vi "Brownian Motion.vi"(7 "Data":T1) -> (0 "Simulation Objects":refnum<class "SimulationObject.lvclass">[](array[class]), 1 "Cell Size":i16, 2 "Gravity Vector out":refnum<class "Vector2.lvclass">, 3 "Background Color out":u32(colorbox))   [LabVIEW 2022 SP3]
uses:
  Engine/Math/Vector2/Vector2.lvclass
  Engine/Objects/SimulationObject/SimulationObject.lvclass
  Engine/Objects/SimulationObject/SimulationObject.lvclass/SimulationObject.ctl
  Engine/Objects/Components/PhysicsComponent/PhysicsComponent.lvclass/PhysicsComponent.ctl
  Engine/Math/Vector2/Vector2.lvclass/Vector2.ctl
  <vilib>/numeric/Random Number (Range) I64.vi
  Engine/Math/Vector2/Read x.vi
  Engine/Math/Vector2/Read y.vi
  <vilib>/numeric/sub_Random U32.vi
  Engine/Objects/Shapes/CircleShape/CircleShape.lvclass
  D:/Programowanie/Studia/Labview/CollisionSimulator/Project/Engine/Objects/Shapes/Shapeable/Shapeable.lvclass
  Engine/Objects/Components/PhysicsComponent/PhysicsComponent.lvclass
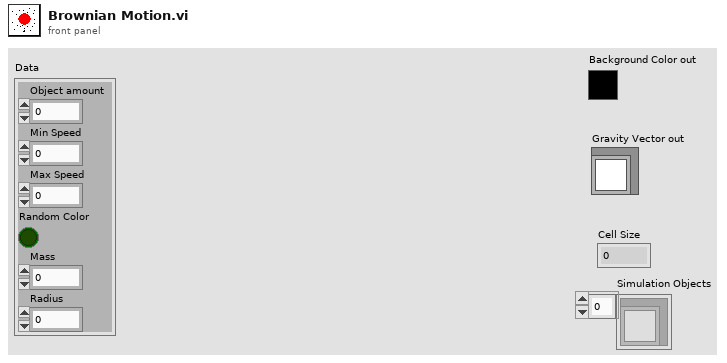
[diagram p1: front panel]
types:
  T1 = cluster{"Object amount":i16, "Min Speed":dbl, "Max Speed":dbl, "Random Color":bool, "Mass":dbl, "Radius":i16}
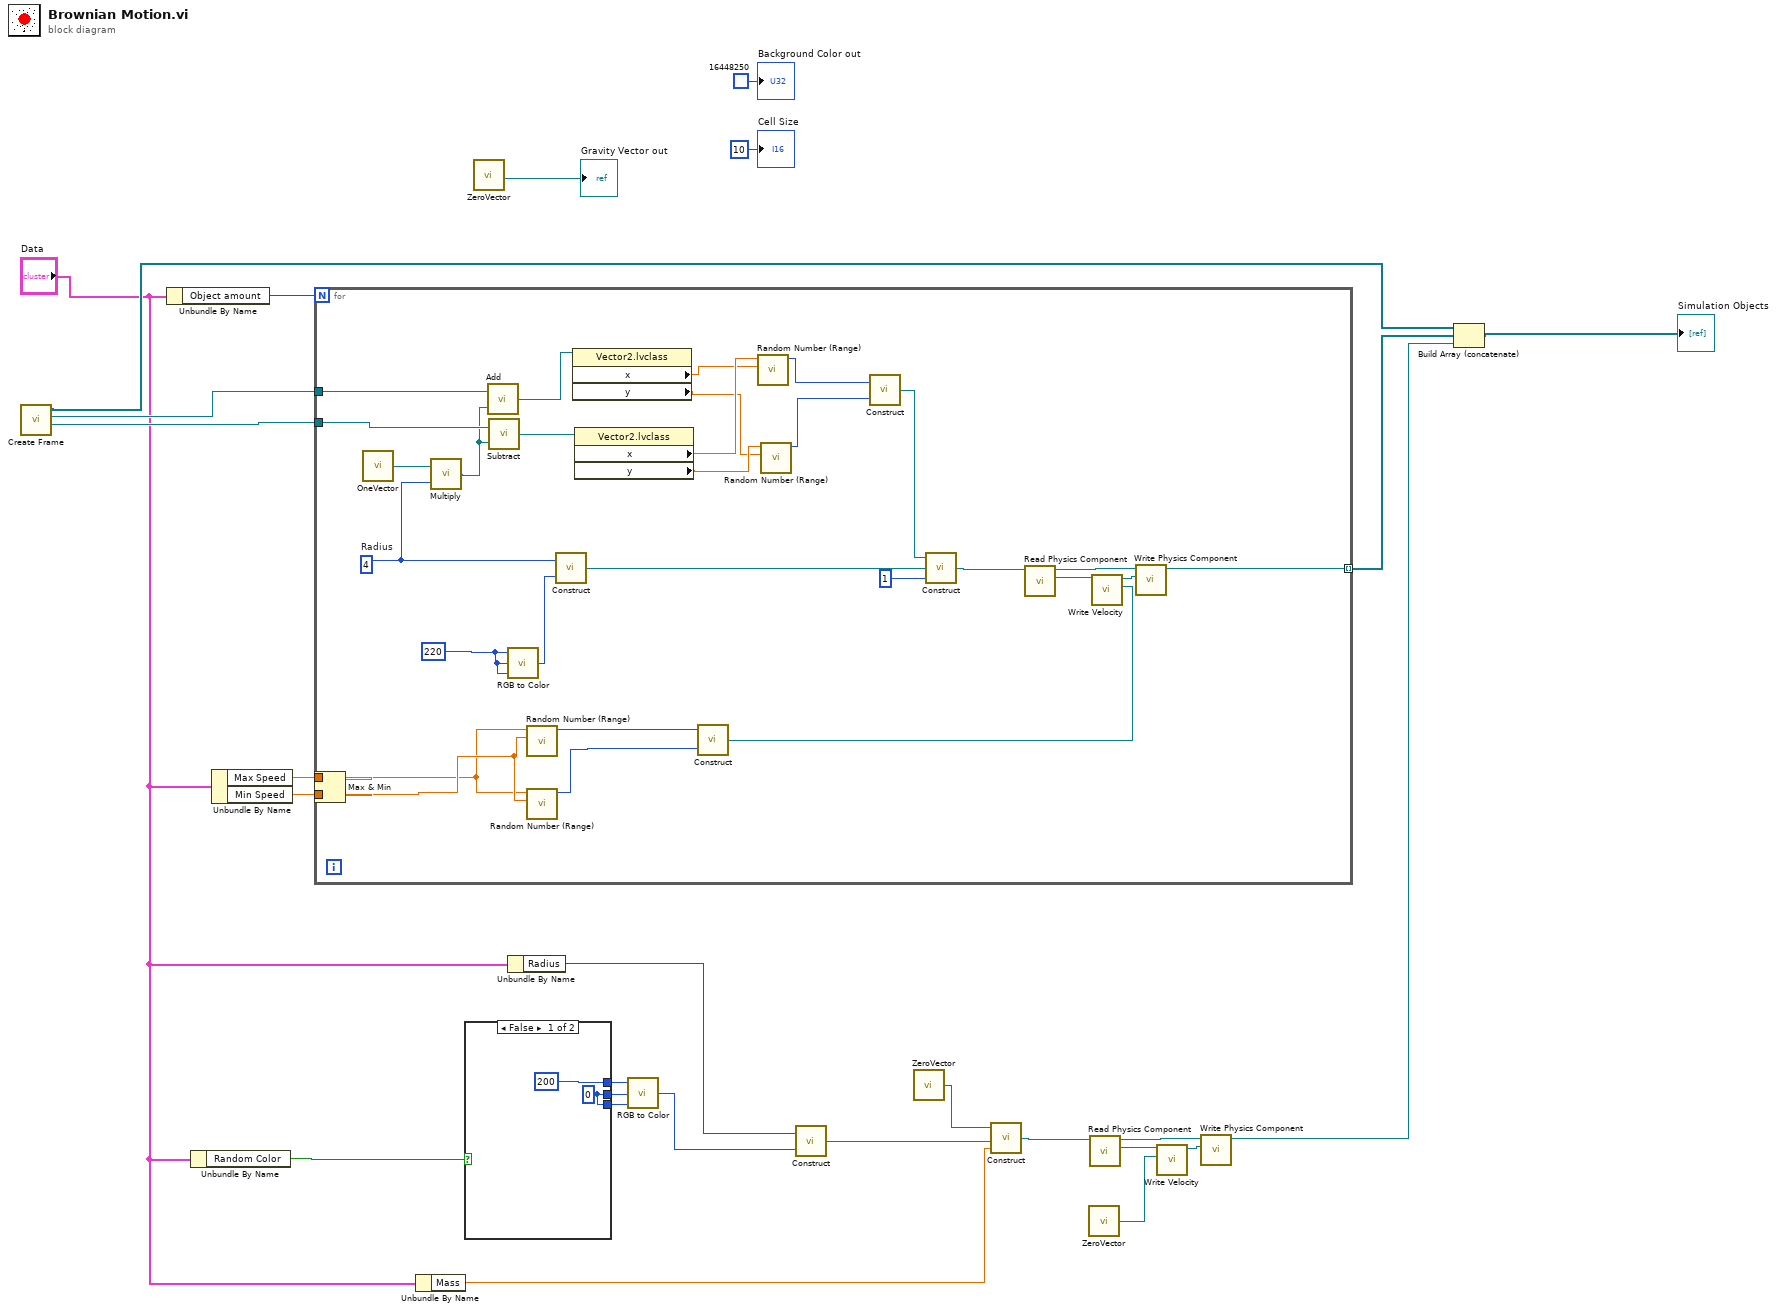
[diagram p0: block diagram]
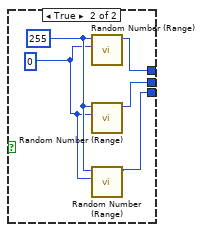
[diagram p2: hidden frame]
diagram:
  n1 = call "Create Frame.vi"() -> ("Max Available Position"=w25:refnum<class "Vector2.lvclass">, "Min Available Position"=w26:refnum<class "Vector2.lvclass">, "Simulation Objects"=w20:refnum<class "SimulationObject.lvclass">[])  [unwired: 4 in, 1 out]
  n2 = Unbundle By Name("Data") -> ("Object amount"=w27:i16)
  n3 = Unbundle By Name("Data") -> ("Random Color"=w13:bool)
  n4 = Unbundle By Name("Data") -> ("Max Speed"=w24:dbl, "Min Speed"=w23:dbl)
  n5 = Max & Min(x=w24, y=w23) -> (max(x,y)=w22:dbl, min(x,y)=w21:dbl)
  n6 = for {
    N: w27 -> [_]
    tunnel: w26 -> [w39]
    tunnel: w25 -> [w49]
    tunnel: w21 -> [w42]
    tunnel: w22 -> [w41]
    tunnel: [w40] -> w19 mode=indexing
    w30 = u8 220 ("R")
    w48 = 4  # Radius
    n7 = call "OneVector.vi"() -> ("One Vector"=w38:refnum<class "Vector2.lvclass">)
    n8 = call "Multiply.vi"("Scalar"=w48, "Vector in"=w38) -> ("Vector out"=w37:refnum<class "Vector2.lvclass">)
    n9 = call "Add.vi"("Vec2 b in"=w37, "Vec2 a in"=w39) -> ("Vec2 out"=w36:refnum<class "Vector2.lvclass">)
    n10 = call "Subtract.vi"("Vec2 b in"=w37, "Vec2 a in"=w49) -> ("Vec2 out"=w35:refnum<class "Vector2.lvclass">)
    n11 = call <vilib>:"RGB to Color.vi"("B"=w30, "G"=w30, "R"=w30) -> ("Color"=w51:u32)
    n12 = call-poly <vilib>:"Random Number (Range).vi"("lower bound (-100)"=w42, "upper bound (100)"=w41) -> ("number"=w44:i64)  [unwired: 9 in]
    n13 = call-poly <vilib>:"Random Number (Range).vi"("lower bound (-100)"=w42, "upper bound (100)"=w41) -> ("number"=w43:i64)  [unwired: 9 in]
    n14 = call "Construct.vi"("Color"=w51, "Radius"=w48) -> ("CircleShape out"=w50:refnum<class "CircleShape.lvclass">)
    n15 = property class="Vector2.lvclass"(reference=w36) -> ("x"=w33:sgl, "y"=w31:sgl)  [unwired: 1 in, 2 out]
    n16 = property class="Vector2.lvclass"(reference=w35) -> ("x"=w34:sgl, "y"=w32:sgl)  [unwired: 1 in, 2 out]
    n17 = call "Construct.vi"("y"=w43, "x"=w44) -> ("Vec2 out"=w52:refnum<class "Vector2.lvclass">)
    n18 = call-poly <vilib>:"Random Number (Range).vi"("lower bound (-100)"=w33, "upper bound (100)"=w34) -> ("number"=w47:i64)  [unwired: 9 in]
    n19 = call-poly <vilib>:"Random Number (Range).vi"("lower bound (-100)"=w31, "upper bound (100)"=w32) -> ("number"=w46:i64)  [unwired: 9 in]
    n20 = call "Construct.vi"("y"=w46, "x"=w47) -> ("Vec2 out"=w57:refnum<class "Vector2.lvclass">)
    n21 = call "Construct.vi"("Mass"=i64 1 ("number"), "Shape in"=w50, "Local Position in"=w57) -> ("Simulation Object out"=w56:refnum<class "SimulationObject.lvclass">)
    n22 = call "Read Physics Component.vi"("SimulationObject in"=w56) -> ("Physics Component out"=w53:refnum<class "PhysicsComponent.lvclass">, "SimulationObject out"=w55:refnum<class "SimulationObject.lvclass">)  [unwired: 8 in, 1 out]
    n23 = call "Write Velocity.vi"("Velocity in"=w52, "PhysicsComponent in"=w53) -> ("PhysicsComponent out"=w54:refnum<class "PhysicsComponent.lvclass">)  [unwired: 8 in, 1 out]
    n24 = call "Write Physics Component.vi"("PhysicsComponent.lvclass"=w54, "SimulationObject in"=w55) -> ("SimulationObject out"=w40:refnum<class "SimulationObject.lvclass">)  [unwired: 8 in, 1 out]
  }
  n25 = Unbundle By Name("Data") -> ("Mass"=w5:dbl)
  n26 = case shown="False" w13 {
    tunnel: [i64 200 ("number") w62] -> w14
    tunnel: [w58 w61] -> w15
    tunnel: [w58 w60] -> w16
    frame False {
      w58 = i64 0 ("number")
    }
    frame True {
      w63 = 0
      w64 = 255
      n27 = call-poly <vilib>:"Random Number (Range).vi"("lower bound (-100)"=w63, "upper bound (100)"=w64) -> ("number"=w62:i64)  [unwired: 9 in]
      n28 = call-poly <vilib>:"Random Number (Range).vi"("lower bound (-100)"=w63, "upper bound (100)"=w64) -> ("number"=w61:i64)  [unwired: 9 in]
      n29 = call-poly <vilib>:"Random Number (Range).vi"("lower bound (-100)"=w63, "upper bound (100)"=w64) -> ("number"=w60:i64)  [unwired: 9 in]
    }
  }
  n30 = call "ZeroVector.vi"() -> ("Zero Vector"=→"Gravity Vector out":refnum<class "Vector2.lvclass">)
  n31 = Unbundle By Name("Data") -> ("Radius"=w1:i16)
  n32 = call <vilib>:"RGB to Color.vi"("B"=w16, "G"=w15, "R"=w14) -> ("Color"=w6:u32)
  n33 = call "Construct.vi"("Color"=w6, "Radius"=w1) -> ("CircleShape out"=w7:refnum<class "CircleShape.lvclass">)
  n34 = call "ZeroVector.vi"() -> ("Zero Vector"=w8:refnum<class "Vector2.lvclass">)
  n35 = call "Construct.vi"("Mass"=w5, "Shape in"=w7, "Local Position in"=w8) -> ("Simulation Object out"=w9:refnum<class "SimulationObject.lvclass">)
  n36 = call "ZeroVector.vi"() -> ("Zero Vector"=w3:refnum<class "Vector2.lvclass">)
  n37 = call "Read Physics Component.vi"("SimulationObject in"=w9) -> ("Physics Component out"=w12:refnum<class "PhysicsComponent.lvclass">, "SimulationObject out"=w10:refnum<class "SimulationObject.lvclass">)  [unwired: 8 in, 1 out]
  n38 = call "Write Velocity.vi"("Velocity in"=w3, "PhysicsComponent in"=w12) -> ("PhysicsComponent out"=w11:refnum<class "PhysicsComponent.lvclass">)  [unwired: 8 in, 1 out]
  n39 = call "Write Physics Component.vi"("PhysicsComponent.lvclass"=w11, "SimulationObject in"=w10) -> ("SimulationObject out"=w4:refnum<class "SimulationObject.lvclass">)  [unwired: 8 in, 1 out]
  n40 = Build Array (concatenate)(w20, w19, w4) -> (→"Simulation Objects":refnum<class "SimulationObject.lvclass">[])
  "Background Color out" <- u32 16448250 ("Background Color out")
  "Cell Size" <- i16 10 ("Cell Size")
